vi "Unit Test with ETS.vi"() -> ()   [LabVIEW 2018]
uses:
  PicoScope 3000a.lvclass
  PicoScope 3000a.lvclass/PicoScope 3000a.ctl
  LWS SLA-070/Distro/Projects/12170 Luminar LWS Base/Source/PPLs/Oscilloscope.lvlibp/Oscilloscope.lvclass
  <instrlib>/PicoScope/PicoScope.lvlib
  ps3000a.dll
  C:/Projects/LWS SLA-070/Distro/Projects/12170 Luminar LWS Base/Source/PPLs/Oscilloscope.lvlibp/Oscilloscope.lvclass
panel:
  in  "Trigger Settings":T1
  out "sampleTimePicoseconds":i32
  out "Properties Panel":T2 {"Max Total Capture Time Available (sec)" format="%.3p"; "Sample Frequency" format="%.3p"; "Sample Rate" format="%.3p"; "Max Samples Available" format="%.3p"; "Total Capture Time (sec)" format="%.3p"}
  out "time array":i64[](array[numeric])
  in  "noOfSamples 3":u32
  in  "noOfSamples 2":u32
  out "Waveform Graph":waveform(dbl)(graph)
  out "noOfSamples":u32
  out "handle out":i16
  out "error out 3":errorcluster
  out "Buffers (Max or non-aggregated) 2":T3
  out "Min Buffers 2":T4
  out "overflow":i16
  in  "Props":T5={"threshold upper"=2, "upper hyst"=0, "threshold lower"=0, "lower hyst"=0, "channels"=enum."1", "threshold mode"=enum."level"}
  in  "Number of Samples":i32=1000
  in  "Acquisition Settings":T6={"preTriggerSamples"=0, "postTriggerSamples"=1000, "timebase"=1, "Down-Sample Mode"=0, "Down Sample Ratio"=1} {"Down Sample Ratio" min=1 step=1; "Down-Sample Mode" items=["None"=0, "Aggregate"=1, "Decimate"=2, "Average"=4]}
  in  "PicoSeconds":i32
  in  "ETS Mode":u32=1
  in  "Set":bool
  in  "Channel Numbers":u32[](array[numeric])=[0]
  in  "Channel(s) Config":T7(array[cluster])
  out "error out 2":errorcluster
  in  "stop":bool
  out "error out":errorcluster
  in  "error in (no error)":errorcluster
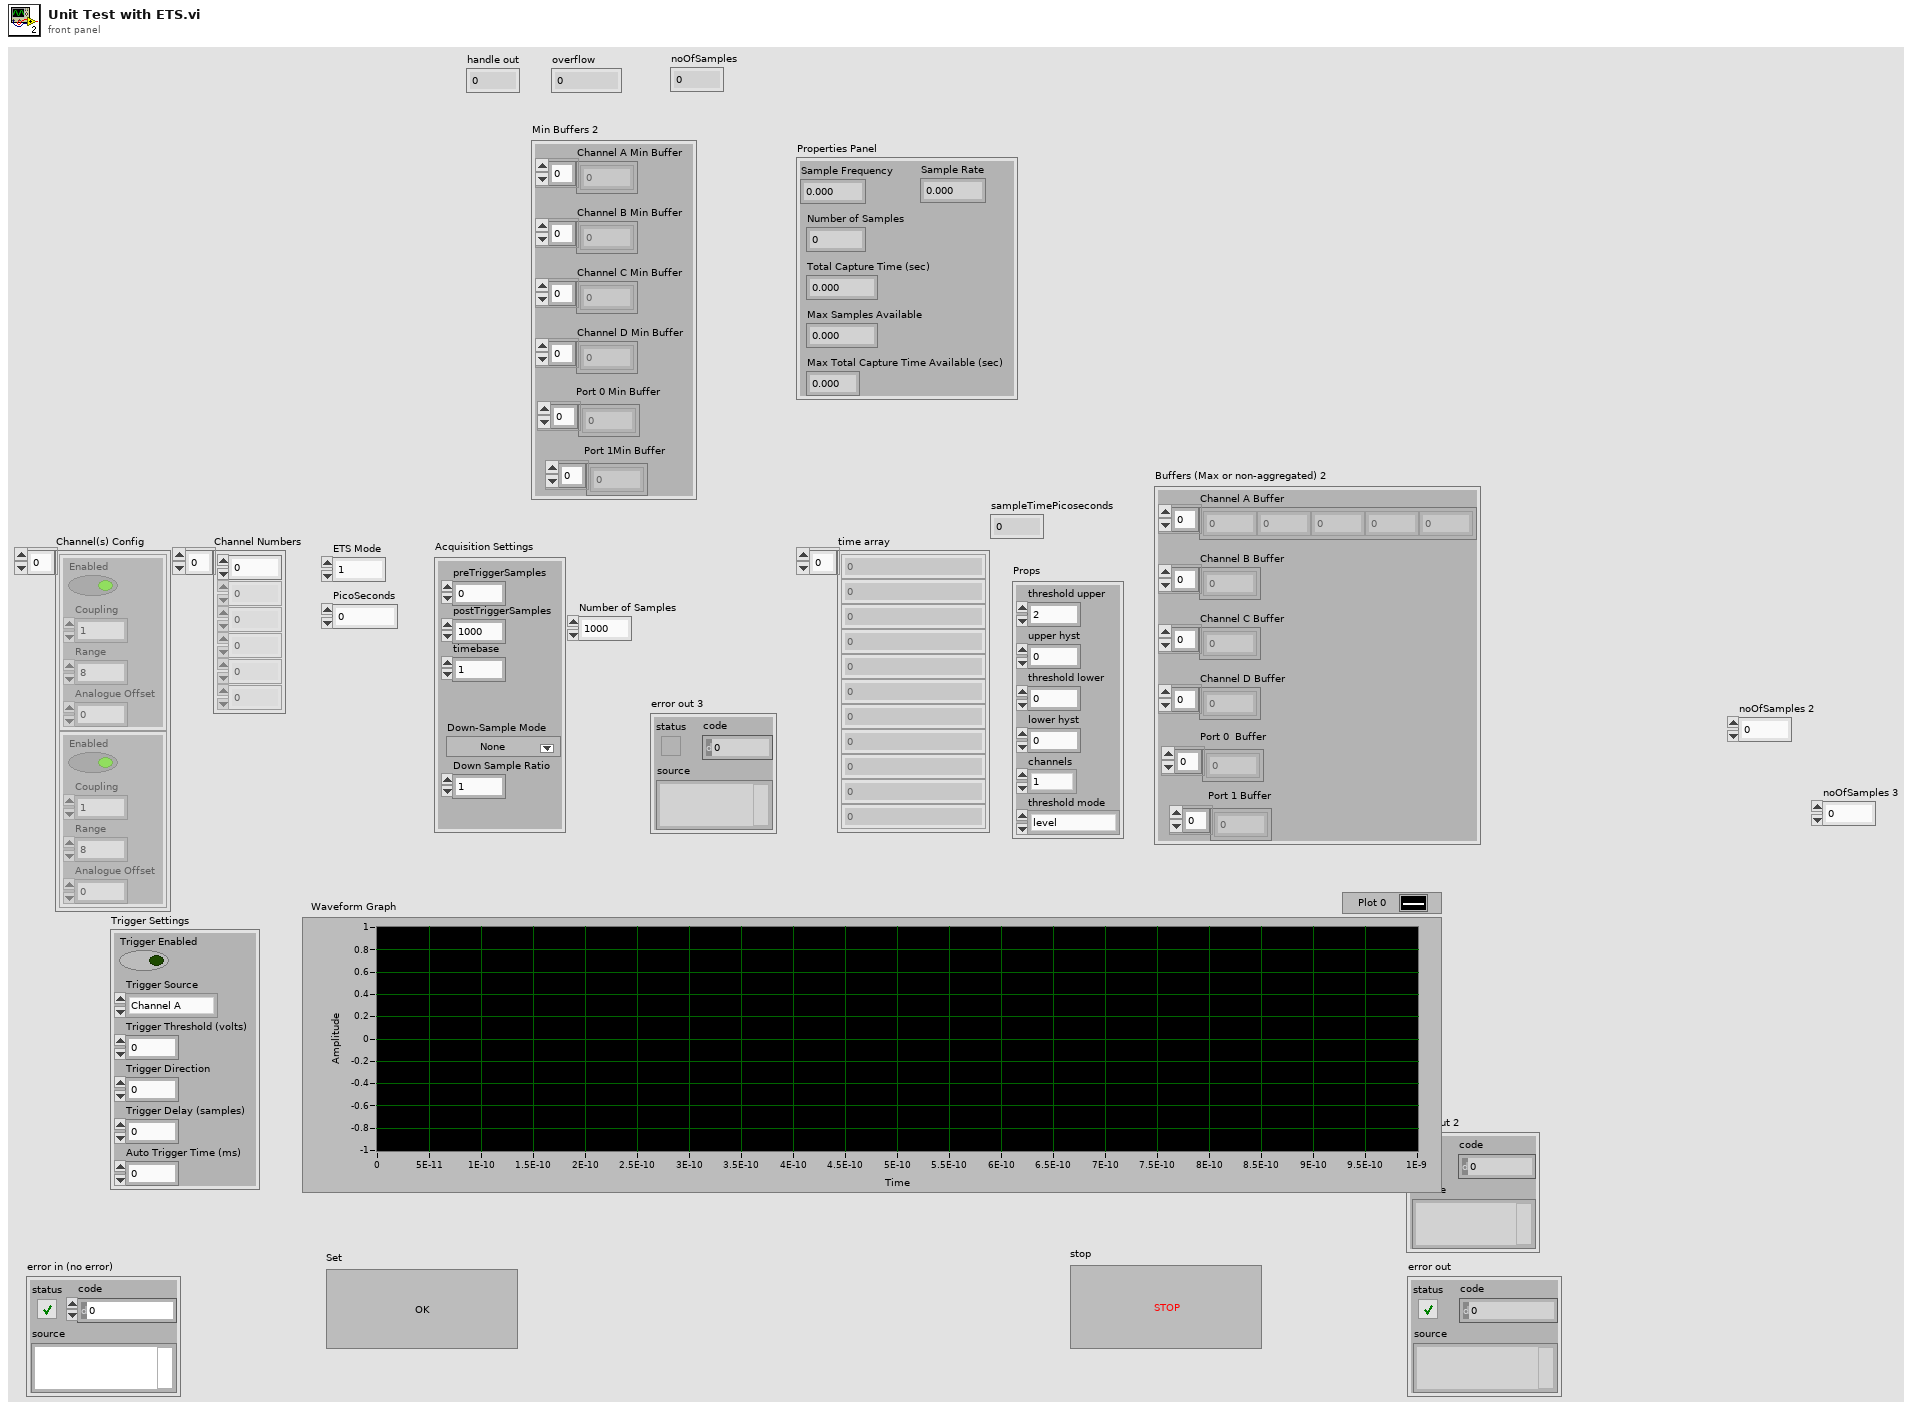
[diagram p1: front panel]
types:
  T1 = cluster{"Trigger Enabled":bool, "Trigger Source":enum32{"Channel A", "Channel B", "Channel C", "Channel D", "Ext."}, "Trigger Threshold (volts)":dbl, "Trigger Direction":u32, "Trigger Delay (samples)":u32, "Auto Trigger Time (ms)":i16}
  T2 = cluster{"Sample Frequency":sgl, "Sample Rate":sgl, "Max Samples Available":i32, "Number of Samples":u32, "Total Capture Time (sec) ":sgl, "Max Total Capture Time Available (sec)":sgl}
  T3 = cluster{"Channel D Buffer":i16[], "Channel C Buffer":i16[], "Channel B Buffer":i16[], "Channel A Buffer":i16[], "Port 0  Buffer ":i16[], "Port 1 Buffer ":i16[]}
  T4 = cluster{"Channel A Min Buffer":i16[], "Channel B Min Buffer":i16[], "Channel C Min Buffer":i16[], "Channel D Min Buffer":i16[], "Port 0 Min Buffer ":i16[], "Port 1Min Buffer ":i16[]}
  T5 = cluster{"threshold upper":i16, "upper hyst":u16, "threshold lower":i16, "lower hyst":u16, "channels":enum16{"1", "2", "3", "4"}, "threshold mode":enum16{"level", "window"}}
  T6 = cluster{"preTriggerSamples":u32, "postTriggerSamples":u32, "timebase":u32, "Down-Sample Mode":i32, "Down Sample Ratio":u32}
  T7 = cluster{"Enabled":bool, "Coupling":u32, "Range":u32, "Analogue Offset":sgl}[]
  T8 = cluster{"Channel A Min Buffer":i16[], "Channel B Min Buffer":i16[], "Channel C Min Buffer":i16[], "Channel D Min Buffer":i16[], "Port 0 Min Buffer":i32[], "Port 1 Min Buffer":i32[]}
  T9 = cluster{"Channel D Buffer":i16[], "Channel C Buffer":i16[], "Channel B Buffer":i16[], "Channel A Buffer":i16[], "Port 0 Max Buffer":i32[], "Port 1 Max Buffer":i32[]}
  T10 = enum32{"Channel A", "Channel B", "Channel C", "Channel D", "Ext."}
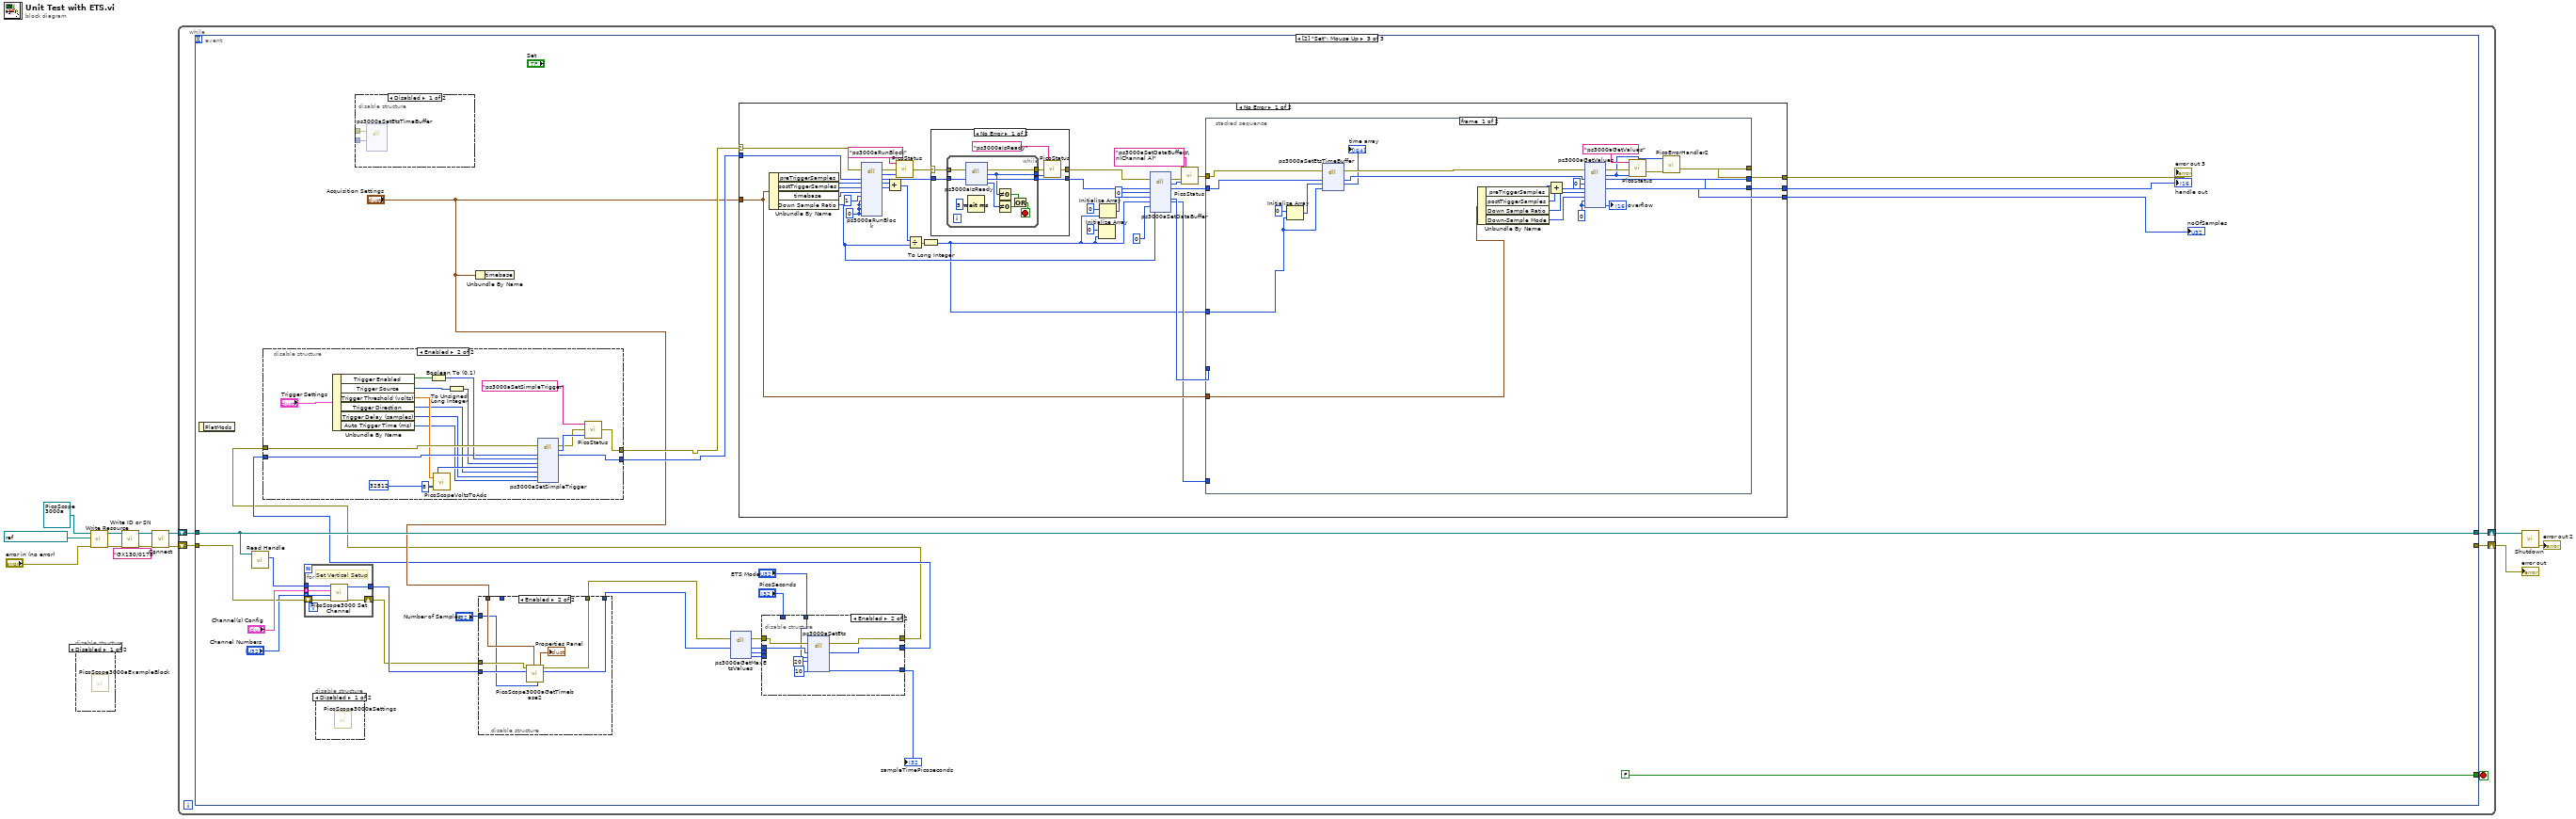
[diagram p0: block diagram]
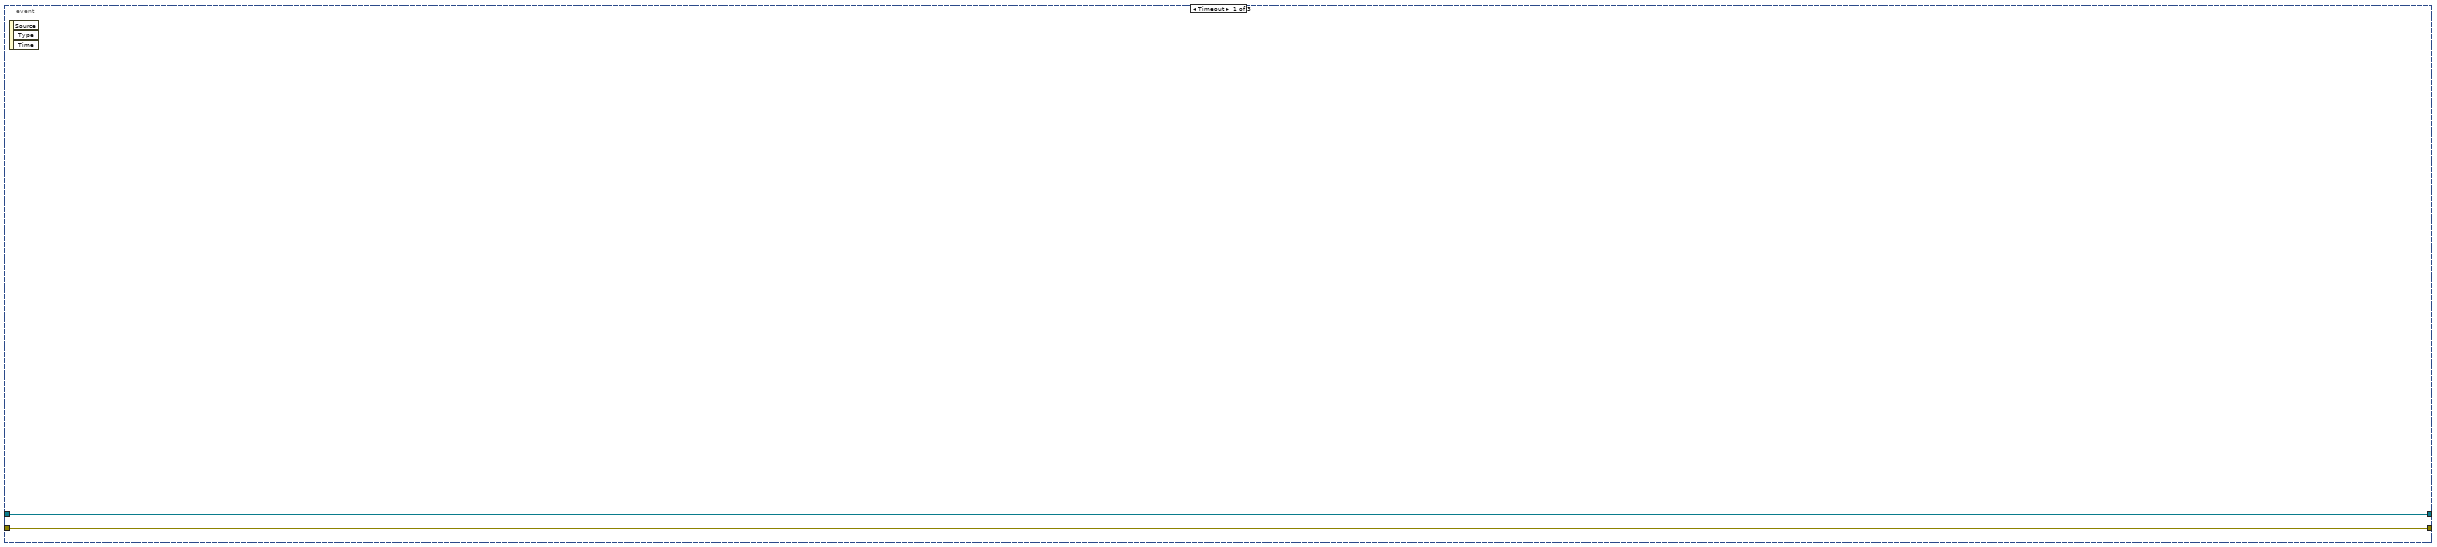
[diagram p3: hidden frame]
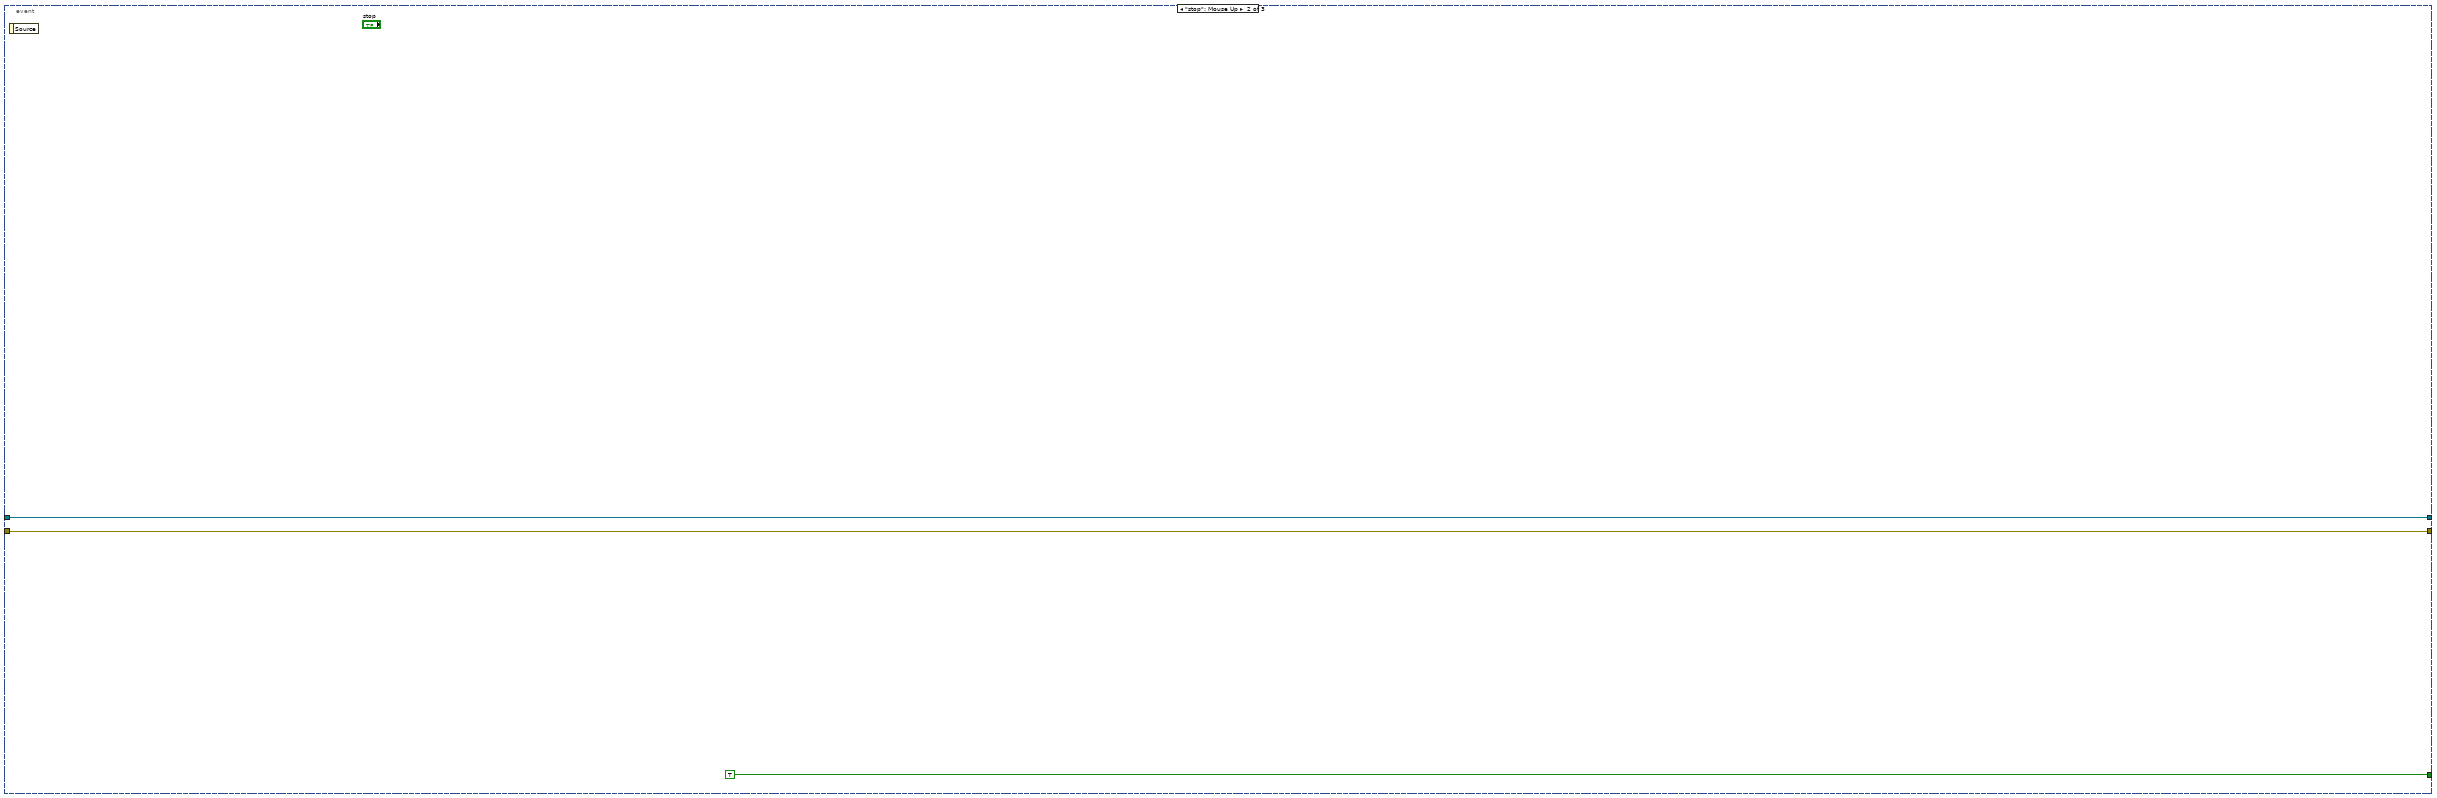
[diagram p4: hidden frame]
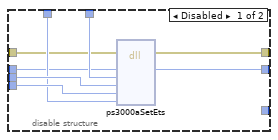
[diagram p6: hidden frame]
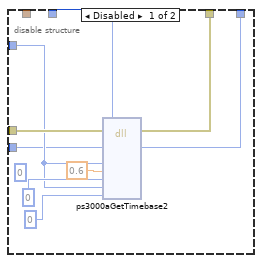
[diagram p7: hidden frame]
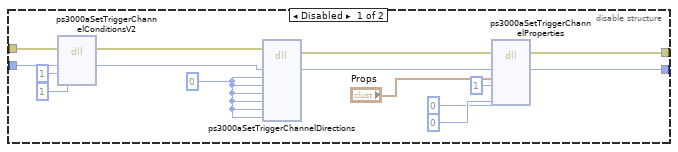
[diagram p8: hidden frame]
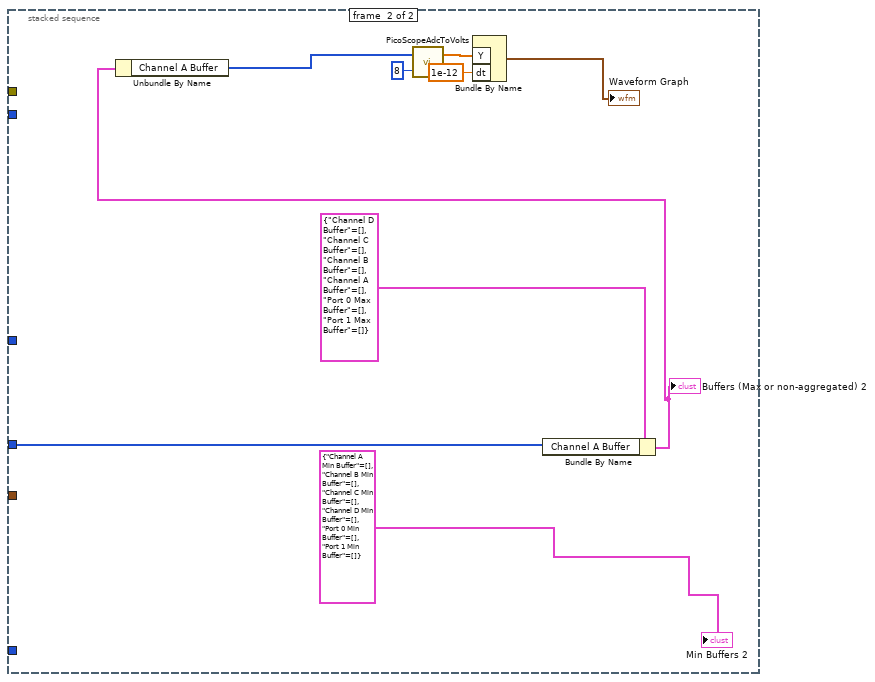
[diagram p9: hidden frame]
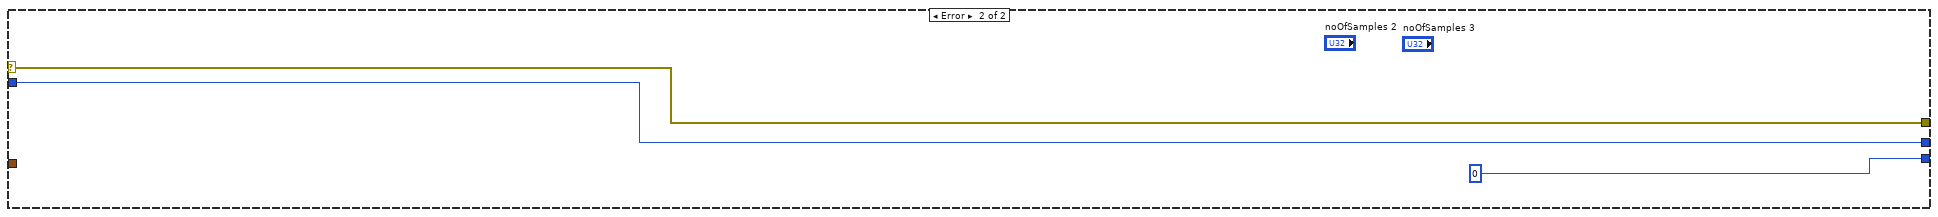
[diagram p11: hidden frame]
diagram:
  n1 = disable-structure shown="Disabled" {
    frame Disabled {
      n2 = call <instrlib>:"PicoScope3000aExampleBlock.vi"() -> ()  [unwired: 1 in]
    }
    frame Enabled {
    }
  }
  n3 = call "Write Resource.vi"("error in (no error)"="error in (no error)", "Resource"=refnum<visa-resource-name> "GX130/0178", "Oscilloscope in"=refnum<class "PicoScope 3000a.lvclass"> refnum ("PicoScope 3000a in")) -> ("error out"=w9:errorcluster, "Oscilloscope out"=w7:refnum<class "PicoScope 3000a.lvclass">)  [unwired: 7 in]
  n4 = call "Write ID or SN.vi"("error in (no error)"=w9, "ID or SN"="GX130/0178", "PicoScope 3000a in"=w7) -> ("error out"=w10:errorcluster, "PicoScope 3000a out"=w8:refnum<class "PicoScope 3000a.lvclass">)  [unwired: 7 in]
  n5 = call-dynamic "Connect.vi"("error in (no error)"=w10, "PicoScope 3000a in"=w8) -> ("error out"=w1:errorcluster, "PicoScope 3000a out"=w2:refnum<class "PicoScope 3000a.lvclass">)  [unwired: 8 in]
  n6 = while {
    shift-right: [w18] -> w13
    shift-left: w2 -> [w17]
    shift-right: [w16] -> w12
    shift-left: w1 -> [w15]
    stop <- w14 stop-if-true
    n7 = event shown="[2] \"Set\": Mouse Up" {
      selector: _ -> [_ _ _]
      dyn-events: _ -> [_ _ _]
      timeout: _ -> [_ _ _]
      tunnel: [w20 w23 w40] -> w18
      tunnel: w17 -> [w20 w23 w40]
      tunnel: [w19 w22 _] -> w16
      tunnel: w15 -> [w19 w22 w47]
      tunnel: [_ TRUE FALSE] -> w14
      event Timeout {
        n8 = event-data() -> ()  [unwired: 1 in, 3 out]
      }
      event "stop": Mouse Up {
        n9 = event-data() -> ()  [unwired: 1 in, 1 out]
      }
      event "Set": Mouse Up {
        n10 = event-data() -> ()  [unwired: 1 in, 1 out]
        n11 = call "Read Handle.vi"("PicoScope 3000a in"=w40) -> ("Handle"=w32:i16)  [unwired: 8 in, 2 out]
        n12 = for {
          tunnel: "Channel(s) Config" -> [w213] mode=indexing
          shift-right: [w212] -> w28
          shift-left: w47 -> [w214]
          tunnel: w32 -> [w211]
          tunnel: "Channel Numbers" -> [w210] mode=indexing
          tunnel: [w209] -> w29
          # "Set Vertical Setup"
          n13 = call <instrlib>:"PicoScope3000 Set Channel.vi"("error in (no error)"=w214, "Channel Settings"=w213, "Channel"=w210, "Handle"=w211) -> ("error out"=w212:errorcluster, "Handle Out"=w209:i16)  [unwired: 5 in, 1 out]
        }
        n14 = disable-structure shown="Disabled" {
          frame Disabled {
            n15 = call <instrlib>:"PicoScope3000aSettings.vi"() -> ()  [unwired: 13 in, 3 out]
          }
          frame Enabled {
          }
        }
        n16 = disable-structure shown="Disabled" {
          disable-tunnel: _ -> [w208 _]
          disable-tunnel: _ -> [w207 _]
          frame Disabled {
            n17 = dll-call lib="ps3000a.dll" fn="ps3000aSetEtsTimeBuffer"(error in=w208, "handle"=w207) -> ()  [unwired: 8 in, 2 out]
          }
          frame Enabled {
          }
        }
        n18 = Unbundle By Name("Acquisition Settings") -> ()  [unwired: 1 out]
        n19 = disable-structure shown="Enabled" {
          disable-tunnel: w28 -> [w74 w80]
          disable-tunnel: [w71 w76] -> w26
          disable-tunnel: "Number of Samples" -> [w70 w77]
          disable-tunnel: _ -> [w69 _]
          disable-tunnel: w29 -> [w67 w81]
          disable-tunnel: "Acquisition Settings" -> [_ w79]
          disable-tunnel: [w66 w75] -> w27
          frame Disabled {
            (unwired) 0 ("TimeIntervalNanoSec")
            n20 = dll-call lib="ps3000a.dll" fn="ps3000aGetTimebase2"(error in=w74, "Handle"=w67, "timebase"=w69, "No Samples"=w70, "TimeIntervalNanoSec"=0.6, "Oversample"=i16 0, "Max Samples"=w70, "Segment Index"=0) -> (error out=w71:errorcluster, "Handle"=w66:i16)  [unwired: 9 in, 1 out]
          }
          frame Enabled {
            n21 = call <instrlib>:"PicoScope3000aGetTimebase2.vi"("Number of Samples"=w77, "Acquisition Settings"=w79, "handle in"=w81, "error in (no error)"=w80) -> ("handle out"=w75:i16, "error out"=w76:errorcluster, "Properties Panel"=→"Properties Panel":T2)  [unwired: 5 in]
          }
        }
        n22 = dll-call lib="ps3000a.dll" fn="ps3000aGetMaxEtsValues"(error in=w26, "Handle"=w27) -> (error out=w41:errorcluster, "Handle"=w33:i16, "Cycles"=w44:i16, "Interleave"=w45:i16)  [unwired: 5 in, 1 out]
        n23 = disable-structure shown="Enabled" {
          disable-tunnel: w45 -> [w57 _]
          disable-tunnel: w44 -> [w56 _]
          disable-tunnel: "ETS Mode" -> [w55 w62]
          disable-tunnel: "PicoSeconds" -> [w54 _]
          disable-tunnel: w41 -> [w53 w65]
          disable-tunnel: [w52 w64] -> w24
          disable-tunnel: [w51 w61] -> w25
          disable-tunnel: w33 -> [w50 w63]
          disable-tunnel: [_ w60] -> w31
          frame Disabled {
            n24 = dll-call lib="ps3000a.dll" fn="ps3000aSetEts"(error in=w53, "Handle"=w50, "ETS Mode"=w55, "Cycles"=w56, "Interleave"=w57, "PicoSeconds"=w54) -> (error out=w52:errorcluster, "Handle"=w51:i16)  [unwired: 7 in, 1 out]
          }
          frame Enabled {
            n25 = dll-call lib="ps3000a.dll" fn="ps3000aSetEts" ("ps3000.dll:_ps3000_open_unit@0")(error in=w65, "handle"=w63, "mode"=w62, "etsCycles"=i16 20, "etsInterleave"=i16 10) -> (error out=w64:errorcluster, "handle"=w61:i16, "sampleTimePicoseconds"=w60:i32)  [unwired: 7 in, 1 out]
          }
        }
        "sampleTimePicoseconds" <- w31
        n26 = disable-structure shown="Enabled" {
          disable-tunnel: w24 -> [w96 w112]
          disable-tunnel: w25 -> [w92 w105]
          disable-tunnel: [w84 w111] -> w36
          disable-tunnel: [w83 w110] -> w35
          frame Disabled {
            w82 = 0 ("CH A")
            n27 = dll-call lib="ps3000a.dll" fn="ps3000aSetTriggerChannelConditionsV2"(error in=w96, "Handle"=w92, "Conditions"=u8 1, "nConditions"=i16 1) -> (error out=w93:errorcluster, "Handle"=w90:i16)  [unwired: 5 in, 1 out]
            n28 = dll-call lib="ps3000a.dll" fn="ps3000aSetTriggerChannelDirections"(error in=w93, "Handle"=w90, "CH A"=w82, "CH B"=w82, "CH C"=w82, "CH D"=w82, "ext"=w82, "aux"=w82) -> (error out=w91:errorcluster, "Handle"=w89:i16)  [unwired: 9 in, 1 out]
            n29 = dll-call lib="ps3000a.dll" fn="ps3000aSetTriggerChannelProperties"(error in=w91, "Handle"=w89, "Props"="Props", "nChannelsProps"=i16 1, "auxoutput enable"=i16 0, "autotrigger millisecs"=0) -> (error out=w84:errorcluster, "Handle"=w83:i16)  [unwired: 7 in, 1 out]
          }
          frame Enabled {
            n30 = Unbundle By Name("Trigger Settings") -> ("Trigger Enabled"=w109:bool, "Trigger Source"=w107:T10, "Trigger Threshold (volts)"=w103:dbl, "Trigger Direction"=w99:u32, "Trigger Delay (samples)"=w98:u32, "Auto Trigger Time (ms)"=w97:i16)
            n31 = Boolean To (0,1)(Boolean=w109) -> (0, 1=w106:i16)
            n32 = call <instrlib>:"PicoScopeVoltsToAdc.vi"("Max_adc"=i16 32512, "Volts"=w103, "Range Index"=u16 8) -> ("ADC count"=w100:i16)
            n33 = To Unsigned Long Integer(number=w107) -> (unsigned 32bit integer=w104:u32)
            n34 = dll-call lib="ps3000a.dll" fn="ps3000aSetSimpleTrigger" ("ps3000.dll:_ps3000_open_unit@0")(error in=w112, "handle"=w105, "enabled"=w106, "source"=w104, "threshold"=w100, "direction"=w99, "delay"=w98, "autoTrigger_ms"=w97) -> (error out=w114:errorcluster, "PICO_STATUS"=w115:u32, "handle"=w110:i16)  [unwired: 8 in, 1 out]
            n35 = call <instrlib>:"PicoStatus.vi"("PICO STATUS"=w115, "error in"=w114, "source"="ps3000aSetSimpleTrigger") -> ("error out"=w111:errorcluster)
          }
        }
        n36 = case shown="No Error" w36 {
          selector: w36 -> [w131 w206]
          tunnel: [w132 w206] -> w39
          tunnel: w35 -> [w130 w205]
          tunnel: [w129 w205] -> w38
          tunnel: [w123 u32 0 ("noOfSamples")] -> w37
          tunnel: "Acquisition Settings" -> [w120 _]
          frame No Error {
            w151 = 0 ("pParameter")
            n37 = Unbundle By Name(w120) -> ("preTriggerSamples"=w141:u32, "postTriggerSamples"=w140:u32, "timebase"=w142:u32, "Down Sample Ratio"=w121:u32)
            n38 = dll-call lib="ps3000a.dll" fn="ps3000aRunBlock" ("ps3000.dll:_ps3000_open_unit@0")(error in=w131, "handle"=w130, "preTriggerSamples"=w141, "postTriggerSamples"=w140, "timebase"=w142, "oversample"=i16 1, "timeindisposed"=w151, "segmentIndex"=w151, "lpReady"=w151, "pParameter"=w151) -> (error out=w138:errorcluster, "PICO_STATUS"=w139:i32, "handle"=w150:i16, "preTriggerSamples"=w148:u32, "postTriggerSamples"=w147:u32)  [unwired: 8 in, 1 out]
            n39 = Add(x=w148, y=w147) -> (x+y=w126:u32)
            n40 = call <instrlib>:"PicoStatus.vi"("PICO STATUS"=w139, "error in"=w138, "source"="ps3000aRunBlock") -> ("error out"=w137:errorcluster)
            n41 = Divide(x=w126, y=w121) -> (x/y=w125:dbl)
            n42 = To Long Integer(number=w125) -> (32bit integer=w117:i32)
            n43 = case shown="No Error" w137 {
              selector: w137 -> [w189 w202]
              tunnel: w150 -> [w191 w203]
              tunnel: [w190 w203] -> w149
              tunnel: [w188 w202] -> w143
              frame No Error {
                n44 = while {
                  tunnel: [w201] -> w190
                  tunnel: w191 -> [w200]
                  tunnel: [w195] -> w186
                  tunnel: w189 -> [w194]
                  tunnel: [w193] -> w187
                  stop <- w199 stop-if-true
                  n45 = dll-call lib="ps3000a.dll" fn="ps3000aIsReady" ("ps3000.dll:_ps3000_open_unit@0")(error in=w194, "handle"=w200) -> (error out=w193:errorcluster, "status"=w195:i32, "handle"=w201:i16, "ready"=w196:i16)  [unwired: 3 in, 1 out]
                  n46 = Wait (ms)(milliseconds to wait=5) -> ()  [unwired: 1 out]
                  n47 = Not Equal To 0?(x=w195) -> (x != 0?=w197:bool)
                  n48 = Not Equal To 0?(x=w196) -> (x != 0?=w198:bool)
                  n49 = Or(x=w197, y=w198) -> (x .or. y?=w199:bool)
                }
                n50 = call <instrlib>:"PicoStatus.vi"("PICO STATUS"=w186, "error in"=w187, "source"="ps3000aIsReady") -> ("error out"=w188:errorcluster)
              }
              frame Error {
              }
            }
            n51 = Initialize Array(i16 0 ("element"), w117) -> ()  [unwired: 1 out]
            n52 = Initialize Array(i16 0 ("element"), w117) -> (w146:i16[])
            n53 = dll-call lib="ps3000a.dll" fn="ps3000aSetDataBuffer" ("ps3000.dll:_ps3000_open_unit@0")(error in=w143, "handle"=w149, "channel"=0, "Buffer"=w146, "bufferLth"=w117, "segmentIndex"=u32 0, "mode"=w121) -> (error out=w135:errorcluster, "PICO_STATUS"=w136:i32, "handle"=w118:i16, "Buffer"=w127:i16[], "bufferLth"=w119:i32)  [unwired: 5 in, 1 out]
            n54 = call <instrlib>:"PicoStatus.vi"("PICO STATUS"=w136, "error in"=w135, "source"="ps3000aSetDataBuffers\n(Channel A)") -> ("error out"=w116:errorcluster)
            n55 = stacked-sequence {
              tunnel: [w170 _] -> w132
              tunnel: [w169 _] -> w129
              tunnel: w127 -> [_ w183]
              tunnel: [w162 _] -> w123
              tunnel: w120 -> [w160 _]
              tunnel: w119 -> [_ _]
              tunnel: w118 -> [w157 _]
              tunnel: w117 -> [w154 _]
              tunnel: w116 -> [w152 _]
              frame #0 {
                w174 = i16 0 ("overflow")
                n56 = Initialize Array(i64 0 ("element"), w154) -> (w155:i64[])
                n57 = dll-call lib="ps3000a.dll" fn="ps3000aSetEtsTimeBuffer"(error in=w152, "handle"=w157, "Buffer"=w155, "BufferLTH"=w154) -> (error out=w159:errorcluster, "handle"=w158:i16, "Buffer"=→"time array":i64[])  [unwired: 4 in, 1 out]
                n58 = Unbundle By Name(w160) -> ("preTriggerSamples"=w165:u32, "postTriggerSamples"=w166:u32, "Down Sample Ratio"=w167:u32, "Down-Sample Mode"=w163:i32)
                n59 = Add(x=w165, y=w166) -> (x+y=w164:u32)
                n60 = dll-call lib="ps3000a.dll" fn="ps3000aGetValues" ("ps3000.dll:_ps3000_open_unit@0")(error in=w159, "handle"=w158, "startIndex"=u32 0, "noOfSamples"=w164, "downSampleRatio"=w167, "downSampleRatioMode"=w163, "segmentIndex"=w174, "overflow"=w174) -> (error out=w173:errorcluster, "PICO_STATUS"=w161:i32, "handle"=w169:i16, "noOfSamples"=w162:u32, "overflow"=→"overflow":i16)  [unwired: 6 in, 1 out]
                n61 = call <instrlib>:"PicoStatus.vi"("PICO STATUS"=w161, "error in"=w173, "source"="ps3000aGetValues") -> ("error out"=w171:errorcluster)
                n62 = call <instrlib>:"PicoErrorHandler2.vi"("error in (no error)"=w171, "handle In"=w161) -> ("error out"=w170:errorcluster)  [unwired: 9 in]
              }
              frame #1 {
                n63 = Bundle By Name(cluster=T9 {"Channel D Buffer"=[], "Channel C Buffer"=[], "Channel B Buffer"=[], "Channel A Buffer"=[], "Port 0 Max Buffer"=[], "Port 1 Max Buffer"=[]} ("Buffers (Max or non-aggregated)"), "Channel A Buffer"=w183) -> (w182:T9)
                "Buffers (Max or non-aggregated) 2" <- w182
                n64 = Unbundle By Name(w182) -> ("Channel A Buffer"=w179:i16[])
                n65 = call <instrlib>:"PicoScopeAdcToVolts.vi"("Range Index"=u16 8, "Data"=w179) -> ("Data (Volts)"=w181:dbl[])  [unwired: 1 in]
                n66 = Bundle By Name("Y"=w181, "dt"=1e-12) -> (→"Waveform Graph":waveform(dbl))  [unwired: 1 in]
                "Min Buffers 2" <- T8 {"Channel A Min Buffer"=[], "Channel B Min Buffer"=[], "Channel C Min Buffer"=[], "Channel D Min Buffer"=[], "Port 0 Min Buffer"=[], "Port 1 Min Buffer"=[]} ("Min Buffers")
              }
            }
          }
          frame Error {
          }
        }
        "error out 3" <- w39
        "handle out" <- w38
        "noOfSamples" <- w37
      }
    }
  }
  "error out" <- w12
  n67 = call "Shutdown.vi"("Oscilloscope in"=w13) -> ("error out"=→"error out 2":errorcluster)  [unwired: 9 in, 1 out]
